vi "Calibration.vi"(8 "error in (no error)":errorcluster, 11 "VISA resource name":refnum<visa-resource-name>="COM1") -> (0 "error in (no error)":errorcluster, 3 "VISA resource name":refnum<visa-resource-name>)   [LabVIEW 2014, in "AD4212C.lvlib"]
uses:
  AD4212C.lvlib
  Control 2.ctl
panel:
  in  "CAL":bool
  out "Peso de caligracion (g)":dbl=200.0
  in  "stop":bool
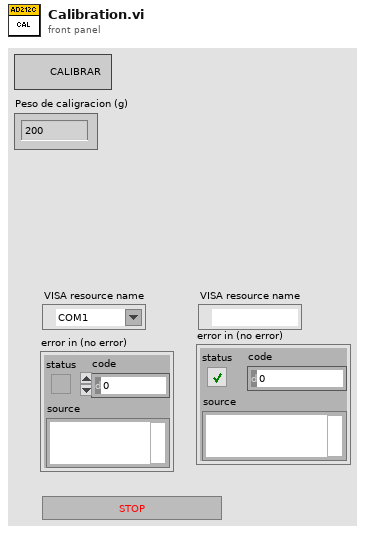
[diagram p1: front panel]
types:
  T1 = typedef "Control 2.ctl" = enum16{"INIT", "CAL", "PRT", "PRT2", "STOP", "READ"}
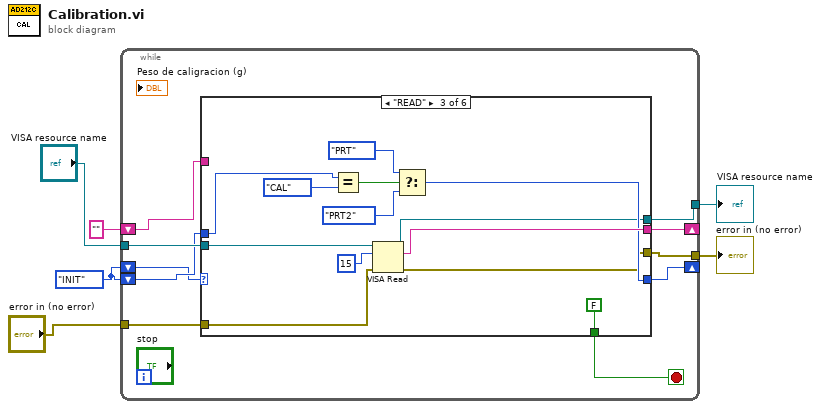
[diagram p0: block diagram]
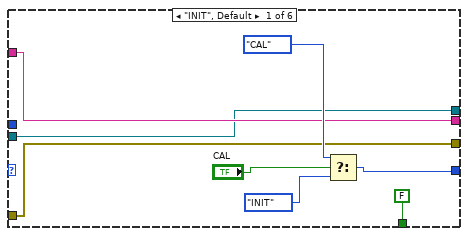
[diagram p2: hidden frame]
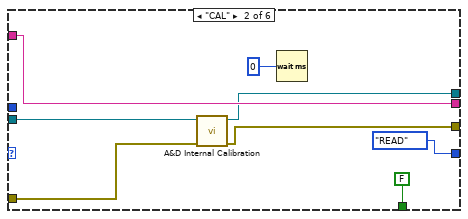
[diagram p3: hidden frame]
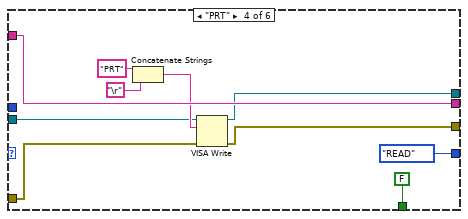
[diagram p4: hidden frame]
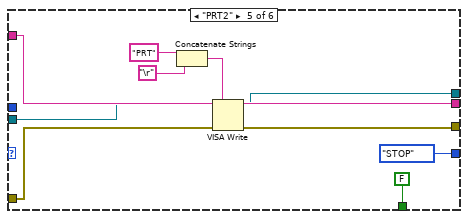
[diagram p5: hidden frame]
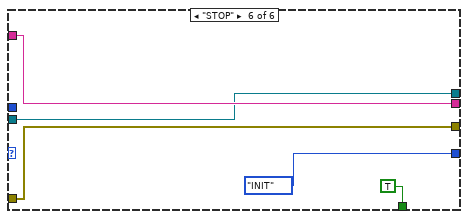
[diagram p6: hidden frame]
diagram:
  w4 = Control_2."INIT"
  n1 = while {
    shift-right: [w16] -> _
    shift-left: w4 -> [w11]
    tunnel: "VISA resource name" -> [w14]
    tunnel: "error in (no error)" -> [w13]
    shift-right: [w7] -> _
    shift-left: "" ("read buffer") -> [w12]
    shift-left: w4 -> [w10]
    tunnel: [w9] -> w1
    tunnel: [w8] -> w2
    stop <- w15 stop-if-true
    n2 = case shown="\"READ\"" w10 {
      tunnel: [w21 Control_2."READ" w39 Control_2."READ" Control_2."STOP" Control_2."INIT"] -> w16
      tunnel: [FALSE FALSE FALSE FALSE FALSE TRUE] -> w15
      tunnel: w14 -> [w18 w30 w45 w49 w60 w67]
      tunnel: w13 -> [w17 w29 w34 w48 w59 w66]
      tunnel: [w19 w27 w44 w54 w64 w69] -> w7
      tunnel: w12 -> [w19 w27 _ w54 w64 w69]
      tunnel: w11 -> [_ _ w43 _ _ _]
      tunnel: [w17 w26 w35 w46 w57 w66] -> w9
      tunnel: [w18 w25 w33 w47 w56 w67] -> w8
      frame "INIT", Default {
        n3 = Select(t=Control_2."CAL", s="CAL", f=Control_2."INIT") -> (s? t:f=w21:T1)
      }
      frame "CAL" {
        n4 = call "A&D Internal Calibration.vi"("error in (no error)"=w29, "VISA resource name"=w30) -> ("error out"=w26:errorcluster, "VISA resource name out"=w25:refnum<visa-resource-name>)  [unwired: 8 in]
        n5 = Wait (ms)(milliseconds to wait=u32 0) -> ()  [unwired: 1 out]
      }
      frame "READ" {
        n6 = Equal?(x=w43, y=Control_2."CAL") -> (x = y?=w41:bool)
        n7 = VISA Read(VISA resource name=w45, byte count=u32 15, error in (no error)=w34) -> (VISA resource name out=w33:refnum<visa-resource-name>, read buffer=w44:string, error out=w35:errorcluster)  [unwired: 1 out]
        n8 = Select(t=Control_2."PRT", s=w41, f=Control_2."PRT2") -> (s? t:f=w39:T1)
      }
      frame "PRT" {
        n9 = Concatenate Strings("PRT" ("Input String"), "\r") -> (w50:string)
        n10 = VISA Write(VISA resource name=w49, write buffer=w50, error in (no error)=w48) -> (VISA resource name out=w47:refnum<visa-resource-name>, error out=w46:errorcluster)  [unwired: 1 out]
      }
      frame "PRT2" {
        n11 = Concatenate Strings("PRT" ("Input String"), "\r") -> (w63:string)
        n12 = VISA Write(VISA resource name=w60, write buffer=w63, error in (no error)=w59) -> (VISA resource name out=w56:refnum<visa-resource-name>, error out=w57:errorcluster)  [unwired: 1 out]
      }
      frame "STOP" {
      }
    }
  }
  "VISA resource name" <- w2
  "error in (no error)" <- w1
